vi "Field of View Conversion.vi"(5 "Pixel Count":dbl, 6 "Field Size (5-255)":dbl) -> (1 "Microns per pixel":dbl, 2 "Field of View (um)":dbl)   [LabVIEW 2020]
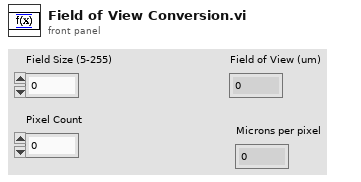
[diagram p1: front panel]
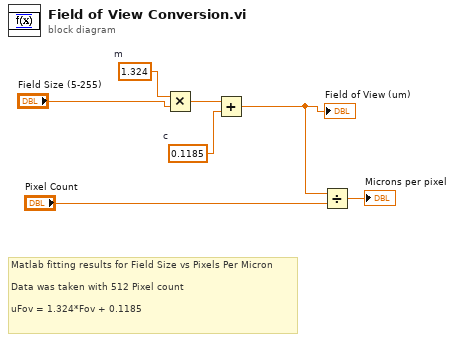
[diagram p0: block diagram]
diagram:
  w5 = 0.1185  # c
  w7 = 1.324  # m
  # "Matlab fitting results for Field Size vs Pixels Per Micron\n\nData was taken with 512 Pixel count\n\nuFov = 1.324*Fov + 0.1185"
  n1 = Multiply(x=w7, y="Field Size (5-255)") -> (x*y=w6:dbl)
  n2 = Add(x=w6, y=w5) -> (x+y=w1:dbl)
  "Field of View (um)" <- w1
  n3 = Divide(x=w1, y="Pixel Count") -> (x/y=→"Microns per pixel":dbl)
